vi "[GlobVar]SensorState.vi"() -> ()   [LabVIEW 2018]
uses:
  TypeDef/ControllerState.ctl
panel:
  in  "Flow_Counter_Offset":u64
  out "target-temp":dbl
  out "target-volume":dbl
  out "State RQST":T1
  out "State Current":T1
  in  "Flow_Counter":u64
  out "DistanceSwitch-5 (Kaffeetasse)":bool
  out "Switch-2 (Lichtschranke)":bool
  out "Switch-4 (Wartungsklappe)":bool
  out "Switch-3 (Tür Hinten)":bool
  out "LevelSwitch-1":bool
  in  "Current Volume (ml)":dbl
  out "PumpVolume_Reached":bool
  out "PumpPressure_Reached":bool
  out "HeaterTemp_Reached":bool
  in  "Pump_ON":bool
  in  "Ventil_OPEN":bool
  in  "Heater_ON":bool
  in  "Current Pressure (psi)":dbl
  in  "Stop":bool
  in  "Current Temp":dbl
  # "Digital Switches"
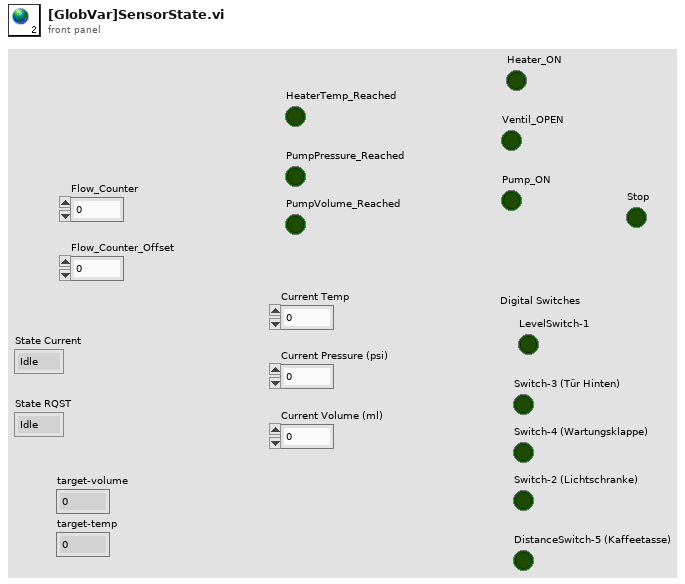
[diagram p1: front panel]
types:
  T1 = typedef "ControllerState.ctl" = enum16{"Idle", "Vorheizen", "Brühen", "Emergency-Stop"}
diagram:
